vi "WiFi HttpsPOST Googlesheet.vi"   [LabVIEW 2014]
uses:
  QwaveSys_ESP8266/QwaveSys_ESP8266.lvlib
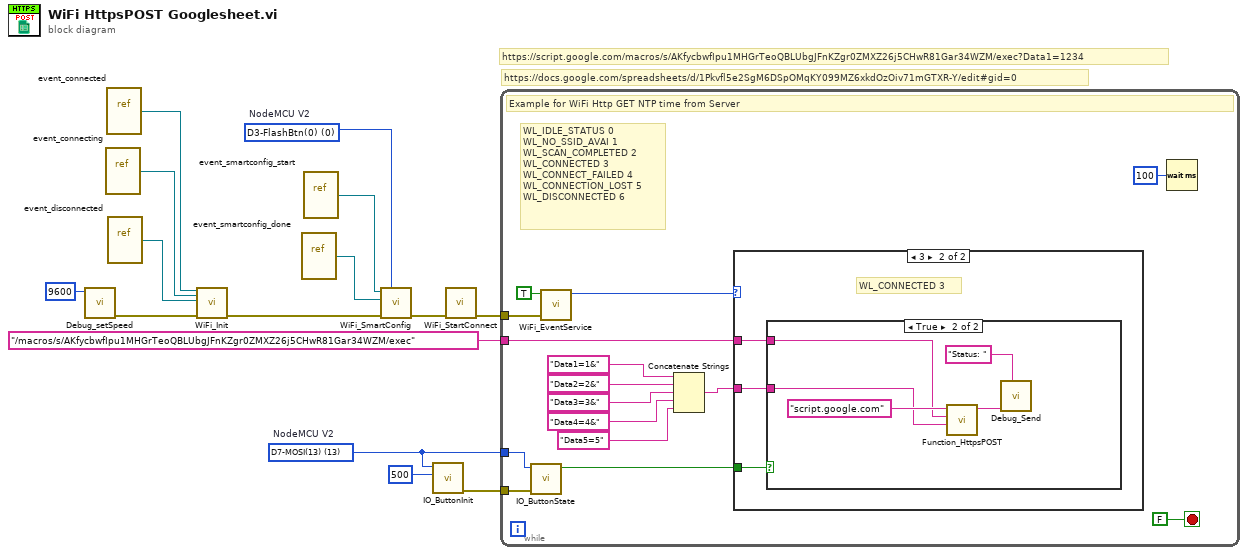
[diagram p0: block diagram]
diagram:
  w2 = u8 13 items=["D0-(LED)-(16)"=16, "D1-SCL(5)"=5, "D2-SDA(4)"=4, "D3-FlashBtn(0)"=0, "D4-(2)"=2, "D5-SCK(14)"=14, "D6-MISO(12)"=12, "D7-MOSI(13)"=13, "D8-SS(15)"=15, "D9-TX(3)"=3, "D10-RX(1)"=1, "ADC0,(17)"=17]  # NodeMCU V2
  w5 = u8 0 items=["D0-(LED)-(16)"=16, "D1-SCL(5)"=5, "D2-SDA(4)"=4, "D3-FlashBtn(0)"=0, "D4-(2)"=2, "D5-SCK(14)"=14, "D6-MISO(12)"=12, "D7-MOSI(13)"=13, "D8-SS(15)"=15, "D9-TX(3)"=3, "D10-RX(1)"=1, "ADC0,(17)"=17]  # NodeMCU V2
  # "https://docs.google.com/spreadsheets/d/1Pkvfl5e2SgM6DSpOMqKY099MZ6xkdOzOiv71mGTXR-Y/edit#gid=0"
  # "https://script.google.com/macros/s/AKfycbwfIpu1MHGrTeoQBLUbgJFnKZgr0ZMXZ26j5CHwR81Gar34WZM/exec?Data1=1234"
  n1 = call "Debug_setSpeed.vi"("Speed"=u32 9600) -> ("error out"=w7:errorcluster)  [unwired: 10 in]
  n2 = vi-ref "event_connecting.vi"() -> (w12:refnum<vi>)
  n3 = vi-ref "event_connected.vi"() -> (w11:refnum<vi>)
  n4 = vi-ref "event_disconnected.vi"() -> (w10:refnum<vi>)
  n5 = call "WiFi_Init.vi"("connected"=w11, "connecting"=w12, "disconnected"=w10, "error in (no error)"=w7) -> ("error out"=w15:errorcluster)  [unwired: 11 in]
  n6 = vi-ref "event_smartconfig_done.vi"() -> (w8:refnum<vi>)
  n7 = vi-ref "event_smartconfig_start.vi"() -> (w9:refnum<vi>)
  n8 = call "WiFi_SmartConfig.vi"("Smart Config Enter Pin"=w5, "error in (no error)"=w15, "smartconfig_done"=w8, "smartconfig_start"=w9) -> ("error out"=w14:errorcluster)  [unwired: 7 in]
  n9 = call "IO_ButtonInit.vi"("debounce (ms)"=u16 500, "PIN"=w2) -> ("error out"=w3:errorcluster)  [unwired: 9 in]
  n10 = call "WiFi_StartConnect.vi"("error in (no error)"=w14) -> ("error out"=w13:errorcluster)  [unwired: 10 in]
  n11 = while {
    tunnel: w13 -> [w29]
    tunnel: w3 -> [w25]
    tunnel: w2 -> [w24]
    tunnel: "/macros/s/AKfycbwfIpu1MHGrTeoQBLUbgJFnKZgr0ZMXZ26j5CHwR81Gar34WZM/exec" -> [w16]
    stop <- FALSE stop-if-true
    # "WL_IDLE_STATUS\t0\nWL_NO_SSID_AVAI\t1\nWL_SCAN_COMPLETED\t2\nWL_CONNECTED\t3\nWL_CONNECT_FAILED\t4\nWL_CONNECTION_LOST\t5\nWL_DISCONNECTED\t6"
    # "Example for WiFi Http GET NTP time from Server"
    n12 = call "IO_ButtonState.vi"("error in (no error)"=w25, "PIN"=w24) -> ("State"=w23:bool)  [unwired: 8 in, 1 out]
    n13 = call "WiFi_EventService.vi"("error in (no error)"=w29, "wait for connected (True)"=TRUE) -> ("Status"=w26:u16)  [unwired: 8 in, 1 out]
    n14 = Concatenate Strings("Data1=1&" ("string"), "Data2=2&" ("string"), "Data3=3&" ("string"), "Data4=4&" ("string"), "Data5=5" ("string")) -> (w17:string)
    n15 = case shown="3" w26 {
      tunnel: w23 -> [_ w33]
      tunnel: w17 -> [_ w32]
      tunnel: w16 -> [_ w31]
      frame 6, Default {
        # "DISCONNECTED or default status"
      }
      frame 3 {
        # "WL_CONNECTED\t3"
        n16 = case shown="True" w33 {
          tunnel: w32 -> [_ w34]
          tunnel: w31 -> [_ w35]
          frame False {
          }
          frame True {
            n17 = call "Function_HttpsPOST.vi"("DATA"=w34, "URI"=w35, "Host"="script.google.com") -> ("Results"=w37:string)  [unwired: 7 in, 1 out]
            n18 = call "Debug_Send.vi"("Name"="Status: ", "DATA"=w37) -> ()  [unwired: 10 in]
          }
        }
      }
    }
    n19 = Wait (ms)(milliseconds to wait=u32 100) -> ()  [unwired: 1 out]
  }
